vi "Set Value.vi"(8 "error in (no error)":errorcluster, 10 "Value":string, 11 "Filled Text Fields in":refnum<class "Filled Text Fields.lvclass">) -> (0 "error out":errorcluster, 3 "Filled Text Fields out":refnum<class "Filled Text Fields.lvclass">)   [LabVIEW 2017, in "Filled Text Fields Actor.lvlib" / "Filled Text Fields.lvclass"]
uses:
  Filled Text Fields.lvclass
  Filled Text Fields.lvclass/Filled Text Fields.ctl
  Data/Data.lvclass/Data.ctl
  Data/setData.vi
  Data/Fire Data Changed.vi
  Data/Data.lvclass
  Filled Text Fields Actor Messages/onValueChange Msg/onValueChange Msg.lvclass
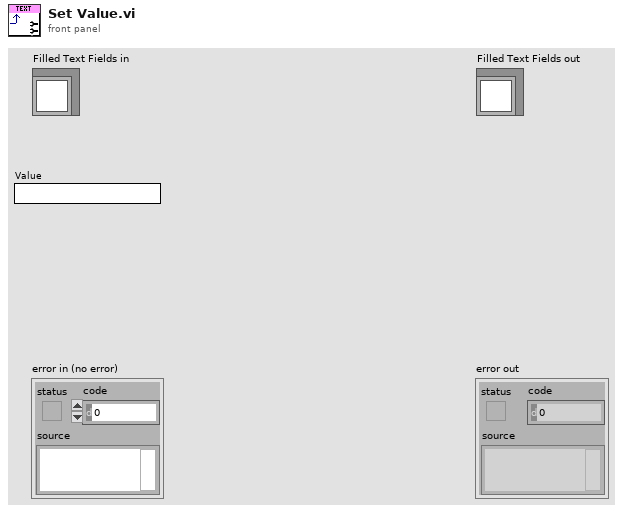
[diagram p1: front panel]
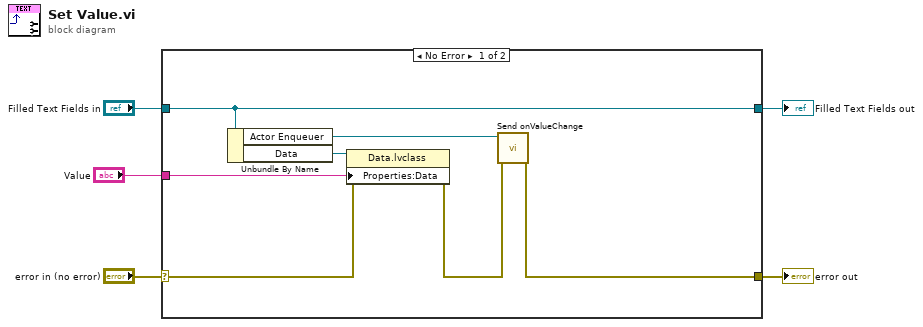
[diagram p0: block diagram]
diagram:
  n1 = case shown="No Error" "error in (no error)" {
    selector: "error in (no error)" -> [w10 w14]
    tunnel: [w6 w14] -> w4
    tunnel: [w12 w13] -> w2
    tunnel: "Filled Text Fields in" -> [w12 w13]
    tunnel: "Value" -> [w9 _]
    frame No Error {
      n2 = Unbundle By Name(w12) -> ("Actor Enqueuer"=w8:refnum<class "Message Enqueuer.lvclass">, "Data"=w11:refnum<class "Data.lvclass">)
      n3 = property class="Data.lvclass"(reference=w11, error in=w10, "Properties:Data"=w9) -> (error out=w7:errorcluster)  [unwired: 1 out]
      n4 = call "Send onValueChange.vi"("error in (no error)"=w7, "Message Enqueuer in"=w8) -> ("error out"=w6:errorcluster)  [unwired: 8 in, 1 out]
    }
    frame Error {
    }
  }
  "error out" <- w4
  "Filled Text Fields out" <- w2
